vi "writeTimestamp.vi"(8 "error in (no error)":errorcluster, 11 "ModbusBuffer in":refnum<class "ModbusBuffer.lvclass">) -> (0 "error out":errorcluster, 3 "ModbusBuffer out":refnum<class "ModbusBuffer.lvclass">)   [LabVIEW 2016, in "RTModbus.lvlib" / "ModbusBuffer.lvclass"]
uses:
  ModbusBuffer.lvclass
  ModbusBuffer.lvclass/ModbusBuffer.ctl
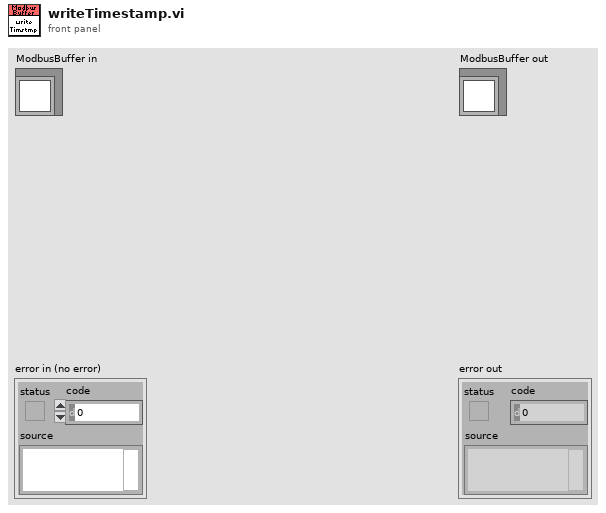
[diagram p1: front panel]
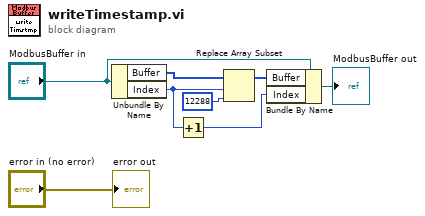
[diagram p0: block diagram]
diagram:
  n1 = Unbundle By Name("ModbusBuffer in") -> ("Buffer"=w8:u16[], "Index"=w4:i32)
  n2 = Increment(x=w4) -> (x+1=w3:i32)
  n3 = Replace Array Subset(array=w8, new element=u16 12288 ("x"), index=w4) -> (w5:u16[])
  n4 = Bundle By Name(cluster="ModbusBuffer in", "Buffer"=w5, "Index"=w3) -> (→"ModbusBuffer out":refnum<class "ModbusBuffer.lvclass">)
  "error out" <- "error in (no error)"
